vi "Fetch Single Record Single Channel(Wfm).vi"(5 "FIFO Type":enum16{"FPGA to Host FIFO (U64)", "Generic"}(ring), 7 "Timeout (s)":i32=5, 8 "error in":errorcluster, 11 "FPGA VI Reference In":refnum<k20>) -> (0 "error out":errorcluster, 2 "Acquired Data":waveform(dbl), 3 "FPGA VI Reference Out":refnum<k20>)   [LabVIEW 2011]
uses:
  <userlib>/FlexRIO Host Library/FlexRIO Host API/Acquire/Fetch/Fetch Acquired Data (U64).vi
  <vilib>/Utility/error.llb/Error Cluster From Error Code.vi
  <vilib>/rvi/errors/niLvFpgaAdjustHostInterfaceError.vi
  <vilib>/rvi/interface/nirviReadWriteControl/nirviReadWriteControl.xnode
  NiFpgaLv.dll
  <vilib>/rvi/interface/Simulation/niFpgaSimulationCallBeginRW.vi
  <userlib>/FlexRIO Host Library/FlexRIO Host Library (User).lvlib
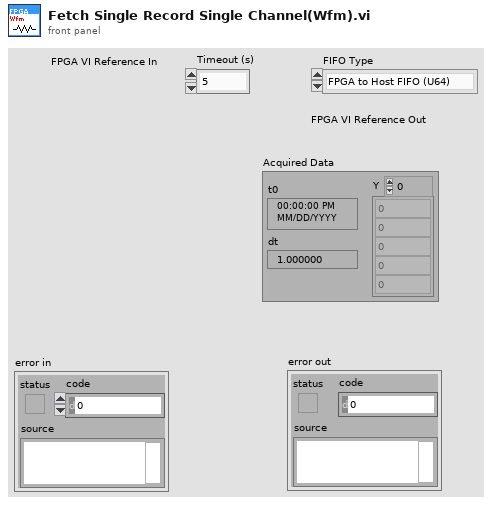
[diagram p1: front panel]
types:
  T1 = cluster{"Load Record Parameters?":bool, "Pre Trigger Samples":u16, "Samples per Record":u16, "Trigger Hold Off":u16, "Record Count":u16}
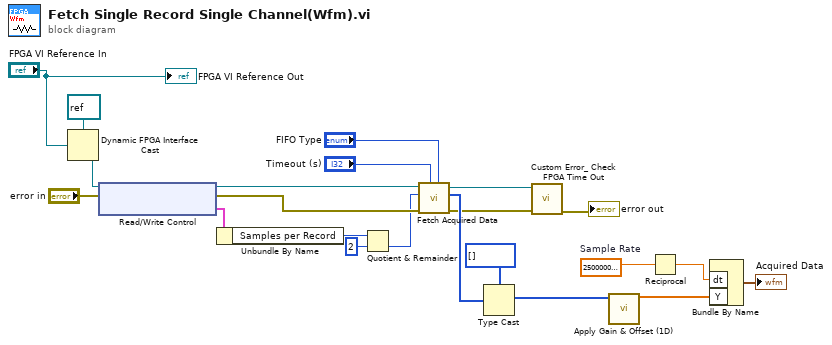
[diagram p0: block diagram]
diagram:
  w4 = 250000000.0  # Sample Rate
  n1 = Dynamic FPGA Interface Cast(Session In=refnum<k20> refnum ("Type"), Type="FPGA VI Reference In") -> (Session Out=w19:refnum<k20>)
  n2 = xnode "Read/Write Control"("FPGA VI Reference In"=w19, "error in"="error in") -> ("FPGA VI Reference Out"=w16:refnum<k20>, "error out"=w15:errorcluster, "Record Parameters"=w18:T1)
  n3 = Unbundle By Name(w18) -> ("Samples per Record"=w17:u16)
  n4 = Quotient & Remainder(x=w17, y=u16 2) -> (floor(x/y)=w5:u16)  [unwired: 1 out]
  n5 = call-poly <userlib>:"Fetch Acquired Data.vi"("FIFO Type"="FIFO Type", "Timeout (s)"="Timeout (s)", "error out"=w15, "Samples"=w5, "FPGA VI Reference In"=w16) -> ("error out"=w9:errorcluster, "Data"=w13:u64[], "FPGA VI Reference Out"=w10:refnum<k20>)  [unwired: 3 in, 1 out]
  n6 = Type Cast(type=i16[] [], x=w13) -> (*(type *) &x=w7:i16[])
  n7 = call <userlib>:"Custom Error_ Check FPGA Time Out.vi"("error in"=w9, "FPGA VI Reference In"=w10) -> ("error out"=→"error out":errorcluster)  [unwired: 8 in, 1 out]
  n8 = call <userlib>:"Apply Gain & Offset (1D).vi"("Raw Data"=w7) -> ("Scaled Data"=w2:dbl[])  [unwired: 10 in]
  n9 = Reciprocal(x=w4) -> (1/x=w3:dbl)
  n10 = Bundle By Name("dt"=w3, "Y"=w2) -> (→"Acquired Data":waveform(dbl))  [unwired: 1 in]
  "FPGA VI Reference Out" <- "FPGA VI Reference In"
